vi "Supply_ComplianceCheck.vi"(8 "error in (no error)":errorcluster, 11 "KE487 in":refnum<class "KE487.lvclass">) -> (0 "error out":errorcluster, 1 "Status string":string, 2 "Compliance exceeded?":bool, 3 "KE487 out":refnum<class "KE487.lvclass">)   [LabVIEW 2018, in "KE487.lvclass"]
uses:
  KE487.lvclass
  SupplyControl.lvclass
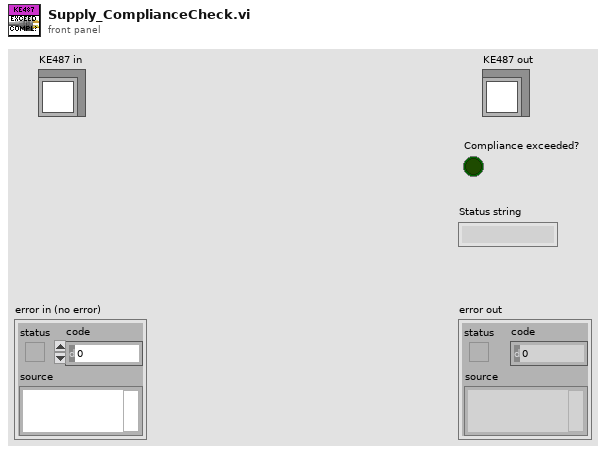
[diagram p1: front panel]
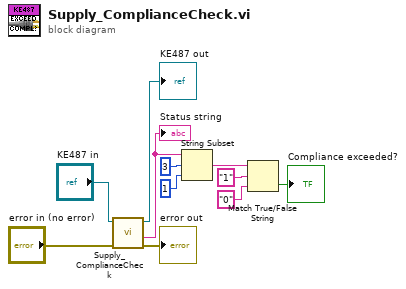
[diagram p0: block diagram]
diagram:
  n1 = call-parent "Supply_ComplianceCheck.vi"("error in (no error)"="error in (no error)", "SupplyControl in"="KE487 in") -> ("error out"=→"error out":errorcluster, "Status string"=w3:string, "SupplyControl out"=→"KE487 out":refnum<class "KE487.lvclass">)  [unwired: 6 in, 1 out]
  "Status string" <- w3
  n2 = String Subset(string=w3, offset (0)=3, length (rest)=1 ("length")) -> (substring=w2:string)
  n3 = Match True/False String(2:"0" ("false string"), 3:"1" ("true string"), 4:w2) -> (0:→"Compliance exceeded?":bool)  [unwired: 1 out]
